vi "PID Turn.vi"(8 "Error In":errorcluster, 9 "Reinitialize":bool, 10 "Target Angle":dbl format="%.2f", 11 "Gyro Angle":dbl) -> (0 "Error Out":errorcluster, 1 "Right Power":dbl, 2 "Left Power":dbl)   [LabVIEW 2016]
uses:
  <vilib>/addons/control/pid/pid.llb/PID (DBL).vi
  <vilib>/addons/control/pid/NI_PID_pid.lvlib
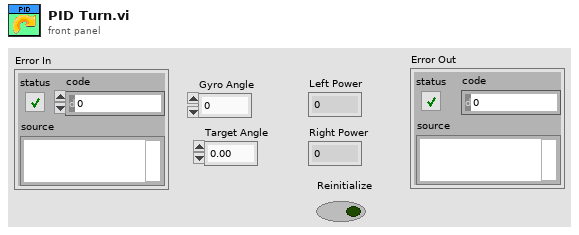
[diagram p1: front panel]
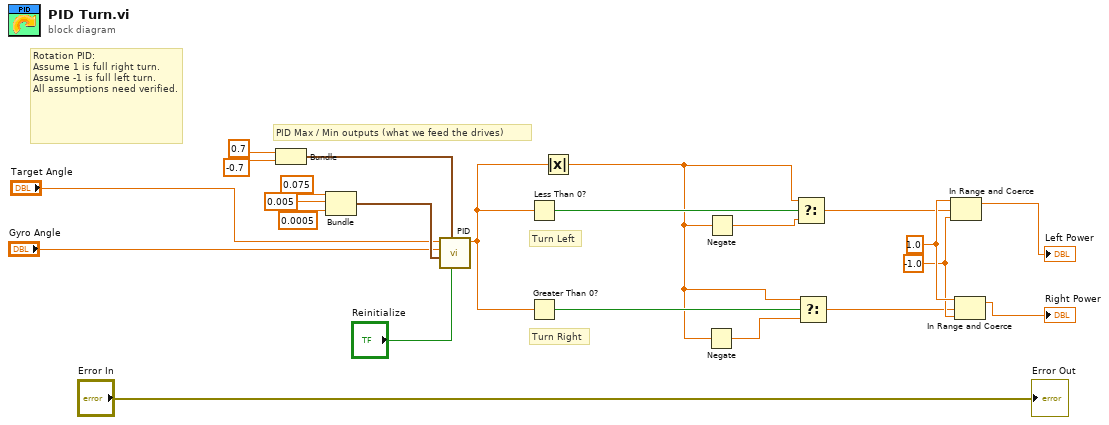
[diagram p0: block diagram]
diagram:
  w11 = -1.0
  w12 = 1.0
  # "Turn Right"
  # "Turn Left"
  # "PID Max / Min outputs (what we feed the drives)"
  # "Rotation PID:\nAssume 1 is full right turn.\nAssume -1 is full left turn.\nAll assumptions need verified."
  n1 = Bundle(0.7, -0.7) -> (w17:cluster{dbl, dbl})  [unwired: 1 in]
  n2 = Bundle(0.075, 0.005, 0.0005) -> (w18:cluster{dbl, dbl, dbl})  [unwired: 1 in]
  n3 = call-poly <vilib>:"PID.vi"("reinitialize? (F)"="Reinitialize", "output range"=w17, "PID gains"=w18, "process variable"="Gyro Angle", "setpoint"="Target Angle") -> ("output"=w6:dbl)  [unwired: 5 in, 1 out]
  n4 = Less Than 0?(x=w6) -> (x < 0?=w10:bool)
  n5 = Greater Than 0?(x=w6) -> (x > 0?=w9:bool)
  n6 = Absolute Value(x=w6) -> (abs(x)=w3:dbl)
  n7 = Negate(x=w3) -> (-x=w1:dbl)
  n8 = Negate(x=w3) -> (-x=w2:dbl)
  n9 = Select(t=w3, s=w10, f=w2) -> (s? t:f=w5:dbl)
  n10 = Select(t=w3, s=w9, f=w1) -> (s? t:f=w4:dbl)
  n11 = In Range and Coerce(upper limit=w12, x=w5, lower limit=w11) -> (coerced(x)=→"Left Power":dbl)  [unwired: 1 out]
  n12 = In Range and Coerce(upper limit=w12, x=w4, lower limit=w11) -> (coerced(x)=→"Right Power":dbl)  [unwired: 1 out]
  "Error Out" <- "Error In"
